vi "Initialize SuBUS Parts.vi"(7 "OVS":u8=16, 8 "Error In":errorcluster, 11 "instrument handle":refnum<k15>) -> (0 "Error Out":errorcluster, 3 "instrument handle out":refnum<k15>)   [LabVIEW 2013]
uses:
  <instrlib>/niHSDIO/niHSDIO.llb/niHSDIO Write Named Waveform (WDT).vi
  <vilib>/Waveform/DWDTOps.llb/DWDT Append Digital Samples.vi
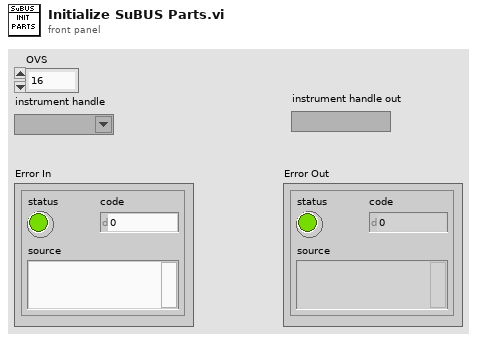
[diagram p1: front panel]
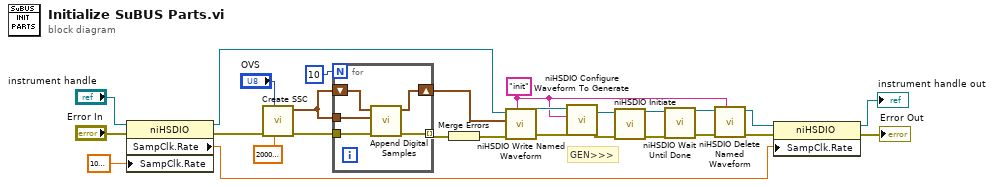
[diagram p0: block diagram]
diagram:
  w19 = "init" ("waveform name (default:\"\")")
  # "GEN>>>"
  n1 = property on="Property Node" class="niHSDIO"(reference="instrument handle", error in="Error In", "SampClk.Rate"=1000000.0 ("sample rate")) -> (reference out=w7:refnum<k15>, error out=w12:errorcluster, "SampClk.Rate"=w4:dbl)
  n2 = call "Create SSC.vi"("sample rate"=20000000.0, "OVS"="OVS", "error in (no error)"=w12) -> ("error out"=w16:errorcluster, "Digital Waveform Graph"=w15:digitalwaveform)  [unwired: 7 in]
  n3 = for {
    N: 10 -> [_]
    shift-right: [w32] -> w1
    shift-left: w15 -> [w31]
    tunnel: w16 -> [w30]
    tunnel: [w29] -> w9 mode=indexing
    tunnel: w15 -> [w28]
    n4 = call-poly <vilib>:"Append Digital Samples.vi"("error in (no error)"=w30, "digital waveform B"=w28, "digital waveform A"=w31) -> ("error out"=w29:errorcluster, "digital waveform out"=w32:digitalwaveform)  [unwired: 7 in]
  }
  n5 = Merge Errors(w9) -> (w8:errorcluster)
  n6 = call-poly <instrlib>:"niHSDIO Write Named Waveform.vi"("waveform name (default:\"\")"=w19, "error in (no error)"=w8, "data"=w1, "instrument handle"=w7) -> ("error out"=w25:errorcluster, "instrument handle out"=w24:refnum<k15>)  [unwired: 6 in]
  n7 = call <instrlib>:"niHSDIO Configure Waveform To Generate.vi"("error in (no error)"=w25, "waveform name"=w19, "instrument handle"=w24) -> ("error out"=w22:errorcluster, "instrument handle out"=w23:refnum<k15>)  [unwired: 7 in]
  n8 = call <instrlib>:"niHSDIO Initiate.vi"("error in (no error)"=w22, "instrument handle"=w23) -> ("error out"=w27:errorcluster, "instrument handle out"=w26:refnum<k15>)  [unwired: 8 in]
  n9 = call <instrlib>:"niHSDIO Wait Until Done.vi"("error in (no error)"=w27, "instrument handle"=w26) -> ("error out"=w21:errorcluster, "instrument handle out"=w20:refnum<k15>)  [unwired: 8 in]
  n10 = call <instrlib>:"niHSDIO Delete Named Waveform.vi"("waveform name (default:\"\")"=w19, "error in (no error)"=w21, "instrument handle"=w20) -> ("error out"=w5:errorcluster, "instrument handle out"=w6:refnum<k15>)  [unwired: 7 in]
  n11 = property on="Property Node" class="niHSDIO"(reference=w6, error in=w5, "SampClk.Rate"=w4) -> (reference out=→"instrument handle out":refnum<k15>, error out=→"Error Out":errorcluster)
